vi "Get Comparison Timestamp.vi"(8 "error in (no error)":errorcluster, 10 "Assert Message":T1, 11 "Assert Build Timestamp Filter in":refnum<class "Assert Build Timestamp Filter.lvclass">) -> (0 "error out":errorcluster, 2 "Comparison Timestamp":timestamp)   [LabVIEW 2016, in "Assert API Components.lvlib" / "Assert Build Timestamp Filter.lvclass"]
uses:
  Assert Build Timestamp Filter.lvclass
  Message Data.ctl
  Failure Actions.ctl
  VI References.ctl
  Assert API Components.lvlib
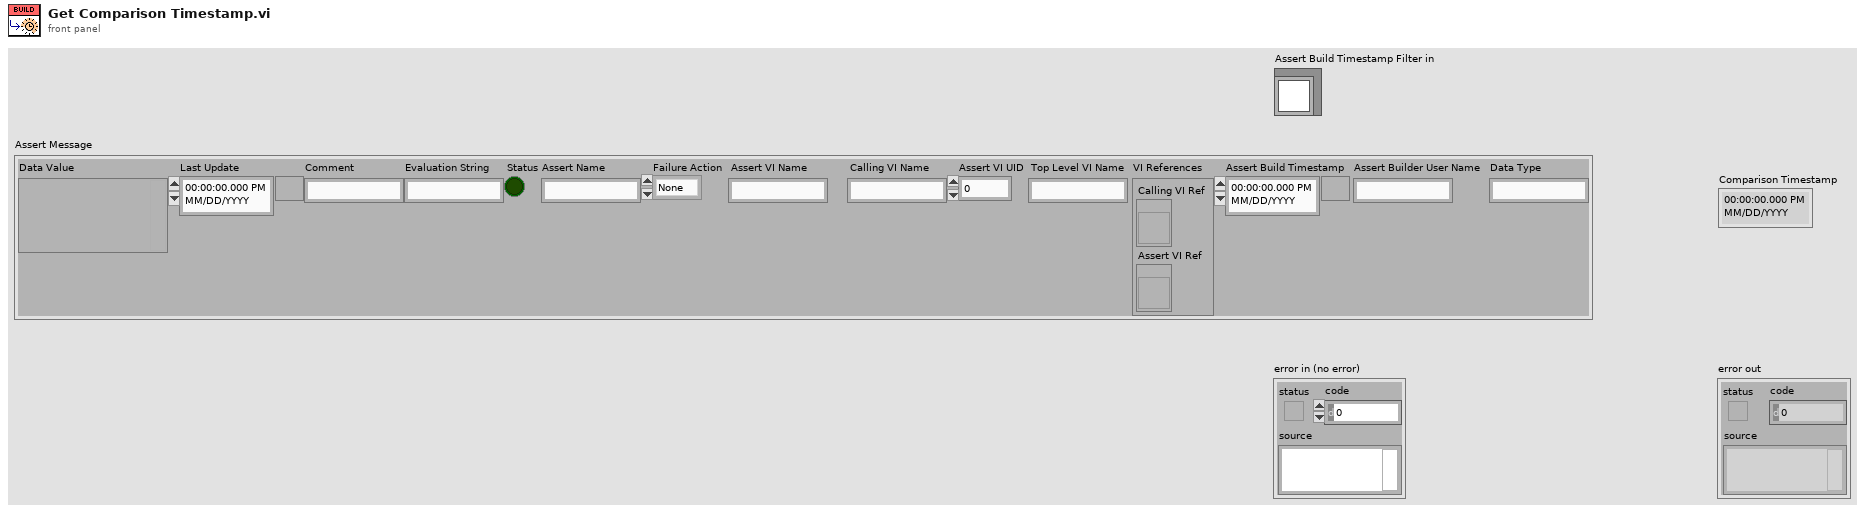
[diagram p1: front panel]
types:
  T1 = typedef "Assert API Components.lvlib/Message Data.ctl" = cluster{"Data Value":variant, "Last Update":timestamp, "Comment":string, "Evaluation String":string, "Status":bool, "Assert Name":string, "Failure Action":T2, "Assert VI Name":string, "Calling VI Name":string, "Assert VI UID":i32, "Top Level VI Name":string, "VI References":T3, "Assert Build Timestamp":timestamp, "Assert Builder User Name":string, "Data Type":string}
  T2 = typedef "Assert API Components.lvlib/Failure Actions.ctl" = enum16{"None", "Log To File", "Pause Execution", "Abort Execution"}
  T3 = typedef "Assert API Components.lvlib/VI References.ctl" = cluster{"Calling VI Ref":refnum<vi>, "Assert VI Ref":refnum<vi>}
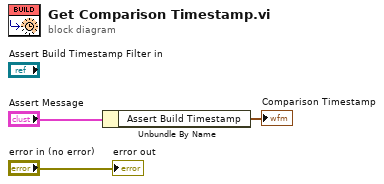
[diagram p0: block diagram]
diagram:
  n1 = Unbundle By Name("Assert Message") -> ("Assert Build Timestamp"=→"Comparison Timestamp":timestamp)
  "error out" <- "error in (no error)"
